vi "Check if SystemLink Feed Exists.vi"(0 "SystemLink repo in":T1, 5 "feed name":string, 11 "error in (no error)":errorcluster) -> (4 "SystemLink repo out":T1, 6 "feed name out":string, 8 "exists?":bool, 15 "error out":errorcluster)   [LabVIEW 2017, in "SystemLink_Repo_API.lvlib"]
doc: "Check if the specified feed exists on the SystemLink repository."
uses:
  SystemLink_Repo_API.lvlib
  <vilib>/httpClient/ClientHandle.ctl
  <vilib>/httpClient/LabVIEWHTTPClient.lvlib
  _support/systemlink repo.ctl
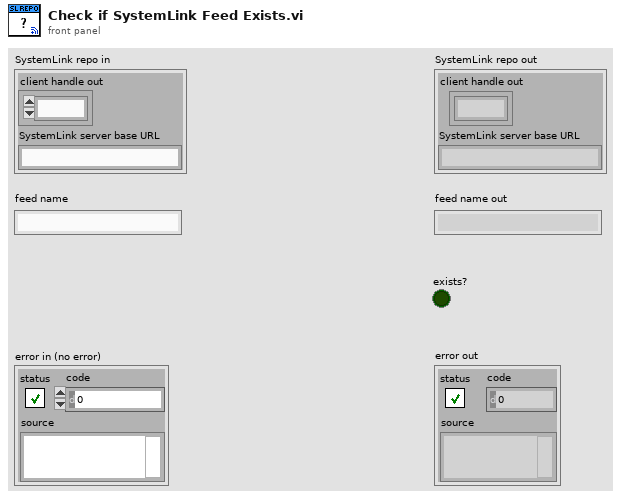
[diagram p1: front panel]
types:
  T1 = typedef "SystemLink_Repo_API.lvlib/systemlink repo.ctl" = cluster{"client handle out":T2, "SystemLink server base URL":string}
  T2 = typedef "LabVIEWHTTPClient.lvlib/ClientHandle.ctl" = refnum<k1>
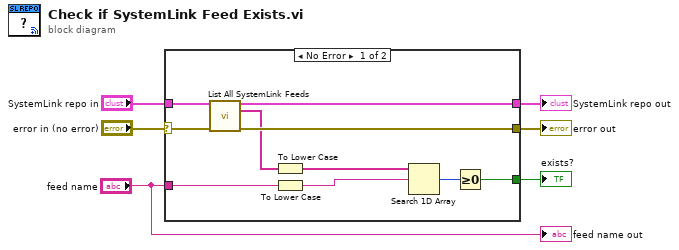
[diagram p0: block diagram]
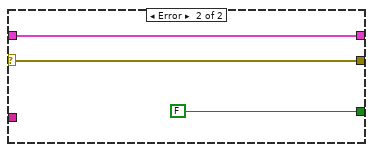
[diagram p2: hidden frame]
diagram:
  n1 = case shown="No Error" "error in (no error)" {
    selector: "error in (no error)" -> [w16 w19]
    tunnel: "SystemLink repo in" -> [w12 w18]
    tunnel: [w13 w19] -> w4
    tunnel: [w11 w18] -> w3
    tunnel: "feed name" -> [w15 _]
    tunnel: [w7 FALSE ("timed out?")] -> w1
    frame No Error {
      n2 = call "List All SystemLink Feeds.vi"("SystemLink repo in"=w12, "error in (no error)"=w16) -> ("SystemLink repo out"=w11:T1, "SystemLink Feed Names"=w10:string[], "error out"=w13:errorcluster)  [unwired: 10 in, 1 out]
      n3 = To Lower Case(string=w10) -> (all lower case string=w9:string[])
      n4 = To Lower Case(string=w15) -> (all lower case string=w8:string)
      n5 = Search 1D Array(1D array=w9, element=w8) -> (index of element=w14:i32)  [unwired: 1 in]
      n6 = Greater Or Equal To 0?(x=w14) -> (x >= 0?=w7:bool)
    }
    frame Error {
    }
  }
  "error out" <- w4
  "SystemLink repo out" <- w3
  "exists?" <- w1
  "feed name out" <- "feed name"
